vi "WPI_CameraIsUSBAddress_EDIT.vi"(8 "error in (no error)":errorcluster, 10 "Enumerate?":bool, 11 "Camera Address In":string="USB 0") -> (0 "error out":errorcluster, 2 "USB?":bool, 3 "Camera Address Out":string)   [LabVIEW 2015]
doc: "Examine the camera address and determine if it is USB or other. If USB, resolve the address and return the ImaqDx addresss string.\n\nThis software is licensed. Open the labview\\readme\\WPI Robotics Library Open Source License.txt file for more information."
uses:
  <vilib>/vision/driver/NI_Vision_Acquisition_Software.lvlib
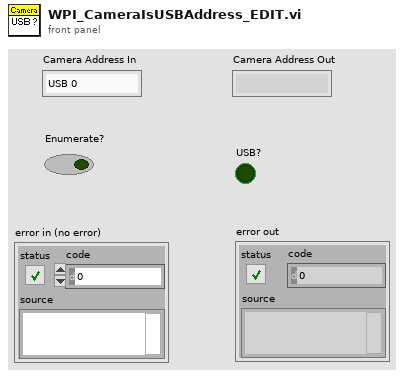
[diagram p1: front panel]
types:
  T1 = cluster{"Type":u32, "Version":u32, "Flags":u32, "SerialNumberHigh":u32, "SerialNumberLow":u32, "BusType":u32, "InterfaceName":string, "VendorName":string, "ModelName":string, "CameraFileName":string, "CameraAttributeURL":string}[]
  T2 = cluster{"Type":u32, "Version":u32, "Flags":u32, "SerialNumberHigh":u32, "SerialNumberLow":u32, "BusType":u32, "InterfaceName":string, "VendorName":string, "ModelName":string, "CameraFileName":string, "CameraAttributeURL":string}
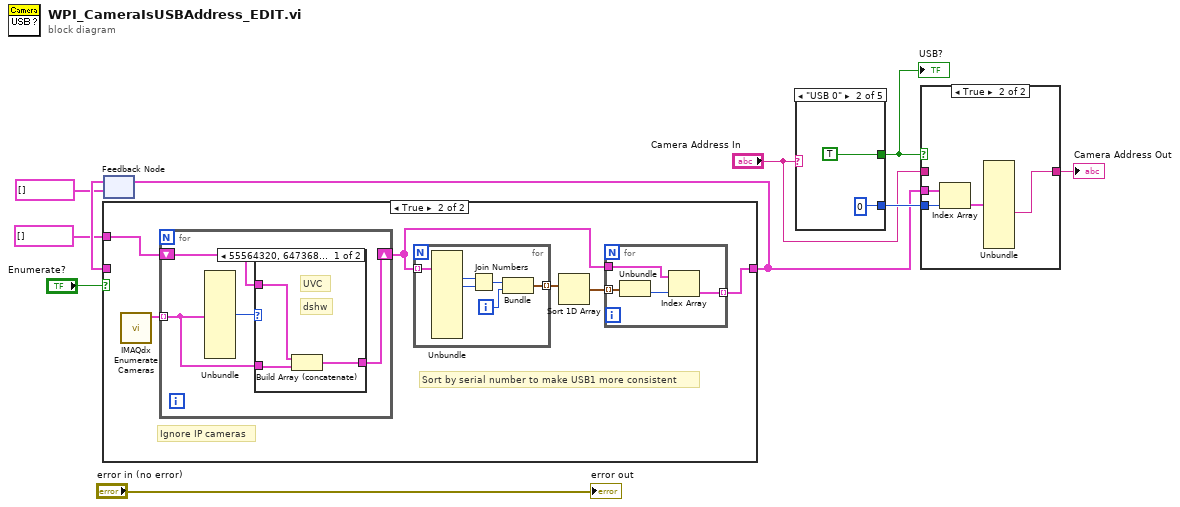
[diagram p0: block diagram]
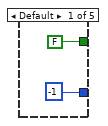
[diagram p5: hidden frame]
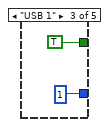
[diagram p6: hidden frame]
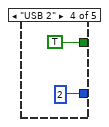
[diagram p7: hidden frame]
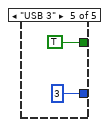
[diagram p8: hidden frame]
diagram:
  n1 = feedback #1(T1 []) -> (w9:T1)
  n2 = case shown="True" "Enumerate?" {
    tunnel: [w11 w15] -> w5
    tunnel: w9 -> [w11 _]
    tunnel: T1 [] -> [_ w12]
    frame False {
    }
    frame True {
      # "Ignore IP cameras"
      # "Sort by serial number to make USB1 more consistent"
      n3 = call <vilib>:"IMAQdx Enumerate Cameras.vi"() -> ("Camera Information Array"=w13:T1)  [unwired: 10 in, 1 out]
      n4 = for {
        shift-right: [w18] -> w14
        shift-left: w12 -> [w19]
        tunnel: w13 -> [w20] mode=indexing
        n5 = Unbundle(w20) -> ("BusType"=w21:u32)  [unwired: 10 out]
        n6 = case shown="55564320, 64736877" w21 {
          tunnel: w20 -> [w23 _]
          tunnel: w19 -> [w24 w25]
          tunnel: [w22 w25] -> w18
          frame 1431716640, 1685284983 {
            # "dshw"
            # "UVC"
            n7 = Build Array (concatenate)(w24, w23) -> (w22:T1)
          }
          frame Default {
          }
        }
      }
      n8 = for {
        tunnel: w14 -> [w35] mode=indexing
        tunnel: [w30] -> w17 mode=indexing
        i -> [w31]
        n9 = Unbundle(w35) -> ("SerialNumberHigh"=w33:u32, "SerialNumberLow"=w34:u32)  [unwired: 9 out]
        n10 = Join Numbers(hi=w33, lo=w34) -> ((hi.lo)=w32:u64)
        n11 = Bundle(w32, w31) -> (w30:cluster{u64, i32})  [unwired: 1 in]
      }
      n12 = Sort 1D Array(array=w17) -> (sorted array=w16:cluster{u64, i32}[])
      n13 = for {
        tunnel: w16 -> [w29] mode=indexing
        tunnel: w14 -> [w27]
        tunnel: [w26] -> w15 mode=indexing
        n14 = Unbundle(w29) -> (w28:i32)  [unwired: 1 out]
        n15 = Index Array(array=w27, index=w28) -> (element=w26:T2)
      }
    }
  }
  n16 = feedback-in #1(w5) -> ()
  n17 = case shown="\"USB 0\"" "Camera Address In" {
    tunnel: [FALSE TRUE TRUE TRUE TRUE] -> w4
    tunnel: [-1 0 1 2 3] -> w6
    frame Default {
    }
    frame "USB 0" {
    }
    frame "USB 1" {
    }
    frame "USB 2" {
    }
    frame "USB 3" {
    }
  }
  "USB?" <- w4
  n18 = case shown="True" w4 {
    tunnel: [w46 w47] -> w7
    tunnel: "Camera Address In" -> [w46 _]
    tunnel: w6 -> [_ w49]
    tunnel: w5 -> [_ w48]
    frame False {
    }
    frame True {
      n19 = Index Array(array=w48, index=w49) -> (element=w50:T2)
      n20 = Unbundle(w50) -> ("InterfaceName"=w47:string)  [unwired: 10 out]
    }
  }
  "Camera Address Out" <- w7
  "error out" <- "error in (no error)"
